vi "Trapezoidal Acceleration.vi"(8 "MaxMotorChangeForward":dbl, 9 "Desired":dbl, 10 "Actual":dbl, 11 "MaxMotorChangeBackward":dbl) -> (1 "In range?":bool, 2 "New Actual":dbl)   [LabVIEW 2015]
doc: "Fixes motor acceleration to a linear rate."
panel:
  in  "AccelRate":dbl
  in  "LoopTime":dbl
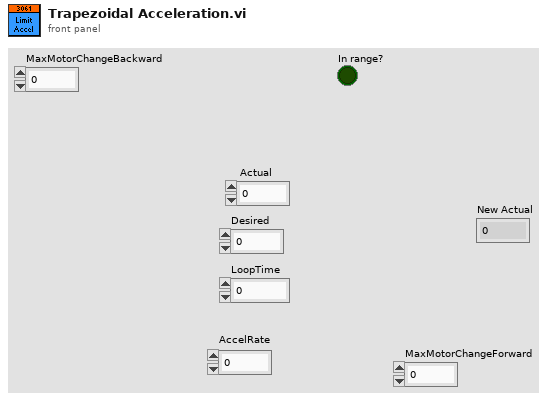
[diagram p1: front panel]
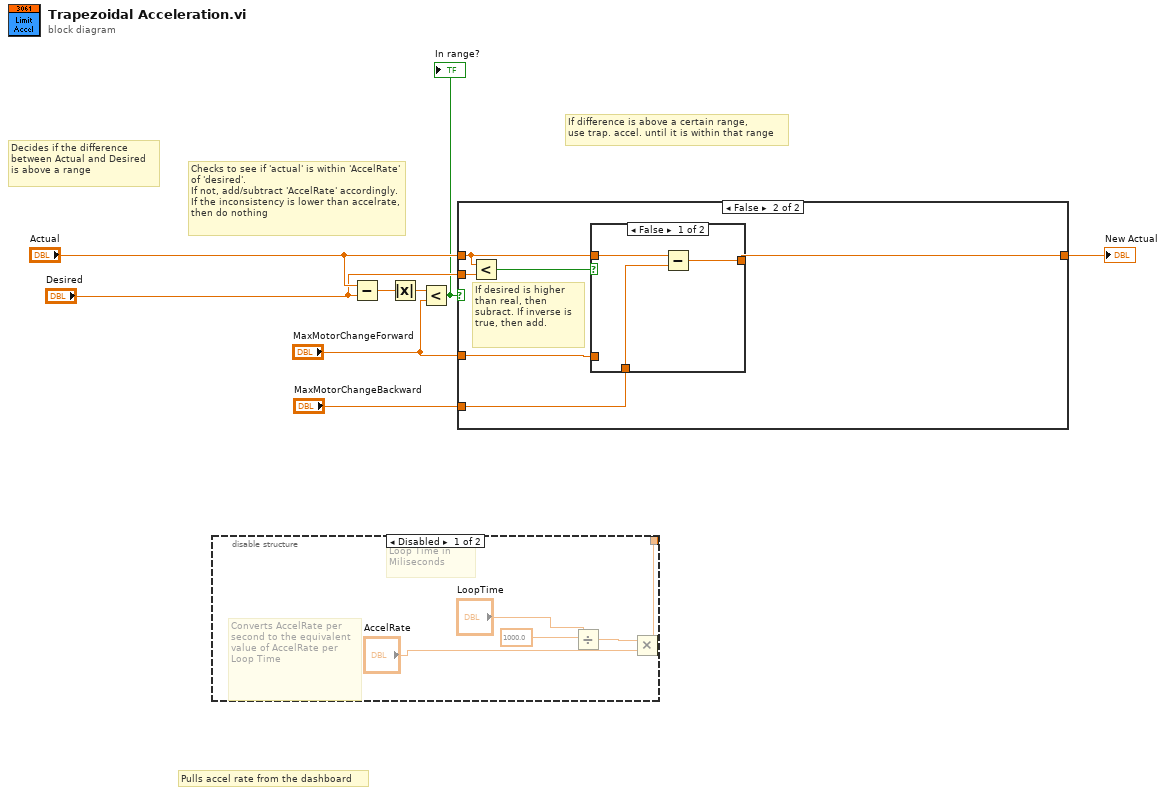
[diagram p0: block diagram]
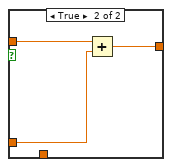
[diagram p4: hidden frame]
diagram:
  # "If difference is above a certain range,\nuse trap. accel. until it is within that range"
  # "Pulls accel rate from the dashboard"
  # "Checks to see if 'actual' is within 'AccelRate' of 'desired'.\nIf not, add/subtract 'AccelRate' accordingly. If the inconsistency is lower than accelrate, then do nothing"
  # "Decides if the difference\nbetween Actual and Desired\nis above a range"
  n1 = disable-structure shown="Disabled" {
    disable-tunnel: [w11 _] -> _
    frame Disabled {
      # "Converts AccelRate per second to the equivalent value of AccelRate per Loop Time"
      # "Loop Time in Miliseconds"
      n2 = Divide(x="LoopTime", y=1000.0) -> (x/y=w12:dbl)
      n3 = Multiply(x=w12, y="AccelRate") -> (x*y=w11:dbl)
    }
    frame Enabled {
    }
  }
  n4 = Subtract(x="Actual", y="Desired") -> (x-y=w4:dbl)
  n5 = Absolute Value(x=w4) -> (abs(x)=w5:dbl)
  n6 = Less?(x=w5, y="MaxMotorChangeForward") -> (x < y?=w3:bool)
  "In range?" <- w3
  n7 = case shown="False" w3 {
    tunnel: [w14 w20] -> w8
    tunnel: "Actual" -> [_ w19]
    tunnel: "Desired" -> [w14 w17]
    tunnel: "MaxMotorChangeForward" -> [_ w16]
    tunnel: "MaxMotorChangeBackward" -> [_ w15]
    frame True {
    }
    frame False {
      # "If desired is higher than real, then subract. If inverse is true, then add."
      n8 = Less?(x=w19, y=w17) -> (x < y?=w18:bool)
      n9 = case shown="False" w18 {
        tunnel: w19 -> [w22 w25]
        tunnel: [w23 w26] -> w20
        tunnel: w16 -> [_ w24]
        tunnel: w15 -> [w21 _]
        frame False {
          n10 = Subtract(x=w22, y=w21) -> (x-y=w23:dbl)
        }
        frame True {
          n11 = Add(x=w25, y=w24) -> (x+y=w26:dbl)
        }
      }
    }
  }
  "New Actual" <- w8
